vi "Gyro Steer.vi"(6 "reinitialize? (F)":bool, 10 "Target Angle":dbl) -> (0 "In Range?":bool, 2 "Steering Out":dbl format="%.2f")   [LabVIEW 2013]
uses:
  Common Code/Change Detect Boolean.vi
  Common Code/Change Detect Double.vi
  Robot Global Data.vi
  <vilib>/addons/control/pid/pid.llb/PID (DBL).vi
  <vilib>/Rock Robotics/WPI/Gyro/WPI_GyroRefNum Registry Get.vi
  <vilib>/Rock Robotics/WPI/Gyro/WPI_GyroGetAngle.vi
  <vilib>/addons/control/pid/NI_PID_pid.lvlib
panel:
  out "PID Output Range":cluster{"output high":dbl, "output low":dbl}
  out "Gyro Angle":dbl
  out "PID Gains":T1
  out "Gyro Error":dbl
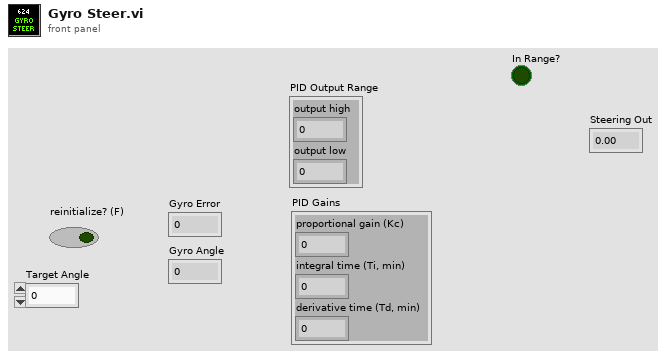
[diagram p1: front panel]
types:
  T1 = cluster{"proportional gain (Kc)":dbl, "integral time (Ti, min)":dbl, "derivative time (Td, min)":dbl}
  T2 = typedef "Dashboard UDP Packet.ctl" = cluster{"Camera":T3, "Gyro":T4, "Encoder":T6, "Auto Shift":T7, "Auton":T8, "Drive/Ramp X":dbl, "Drive/Ramp Y":dbl, "Drive/Battery Cutoff":dbl, "Pressure/Compressor Min Voltage":dbl, "Pressure/Compressor Delay":dbl, "Controller/Strafe Correction":bool, "Shooter":T9, "Rollers":T10, "Abort":bool, "Finish":bool, "IR Halo Sustain Time":dbl, "Disable Compressor":bool, "Center Omni Drive Delay":i32}
  T3 = typedef "Camera Controls.ctl" = cluster{"Camera/View Angle X":dbl, "Camera/Goal Track Timeout":dbl, "Camera/View Angle Y":dbl, "Camera/Goal Exposure":dbl, "Camera/Vision Receive Timeout":dbl, "Camera/Offset 1":dbl, "Camera/Offset 2":dbl}
  T4 = typedef "Gyro Controls.ctl" = cluster{"Gyro/Angle Tolerance":dbl, "Gyro/Steer Closeness Threshold":dbl, "Steer PID":T5, "Steer Close PID":T5}
  T5 = typedef "PID Params.ctl" = cluster{"max":dbl, "min":dbl, "P":dbl, "I":dbl, "D":dbl}
  T6 = typedef "Encoder Controls.ctl" = cluster{"Encoders/Reset":bool, "Encoders/Omni Constant":dbl, "Encoders/Omni Tick Constant":dbl, "Encoders/Left Constant":dbl, "Encoders/Right Constant":dbl, "Encoders/Right Tick Constant":dbl}
  T7 = typedef "Auto Shift Controls.ctl" = cluster{"AutoShift/Upshift Throttle Accel":dbl, "AutoShift/Speed Threshold":dbl, "AutoShift/Upshift Throttle":dbl, "AutoShift/Upshift Accel":dbl, "AutoShift/Downshift Accel":dbl, "AutoShift/Downshift Throttle":dbl, "AutoShift/Delay":dbl, "AutoShift/Enabled":bool}
  T8 = typedef "Auton Controls.ctl" = cluster{"Auton/Left Shoot X-Coord":dbl, "Auton/Right Shoot X-Coord":dbl, "DistDrive/Distance Stop Threshold":dbl, "DistDrive/Max Stop Speed":dbl, "Auton/Back Piston Time":dbl, "Auton/Manual Hot":bool, "Auton/Manual Hot Right":bool, "Default X PID":T5, "Default Y PID":T5}
  T9 = typedef "Shooter Controls.ctl" = cluster{"Shooter/Reset Time":dbl, "Shooter/Release Delay":dbl, "Shooter/Pressure Steady Time":dbl, "Shooter/Misfire Delay":dbl, "Shooter/Ball Settle Time":dbl, "Shooter/Line IR Delay":dbl, "Pressure/Upper PSI Time":dbl, "Pressure/Lower PSI Time":dbl, "Shooter/Punch Delay":dbl, "Shooter/Target Pressure":dbl, "Pressure/Line B":dbl, "Pressure/Line M":dbl, "Pressure/Shooter M":dbl, "Pressure/Shooter B":dbl, "Halo Time":dbl, "Soft Release Delay":dbl, "Soft Unpin Delay":dbl, "Soft Shoot Delay":dbl}
  T10 = typedef "Roller Controls.ctl" = cluster{"Roller/Load IRs Verify Time":dbl, "Roller/Center IR Latch Time":dbl, "Roller/Speed Front":dbl, "Roller/Speed Back":dbl, "Roller/Entry Timeout":dbl, "Roller/To Center Timeout":dbl, "Roller/Sustain Time":dbl, "Roller/Verify Center Time":dbl}
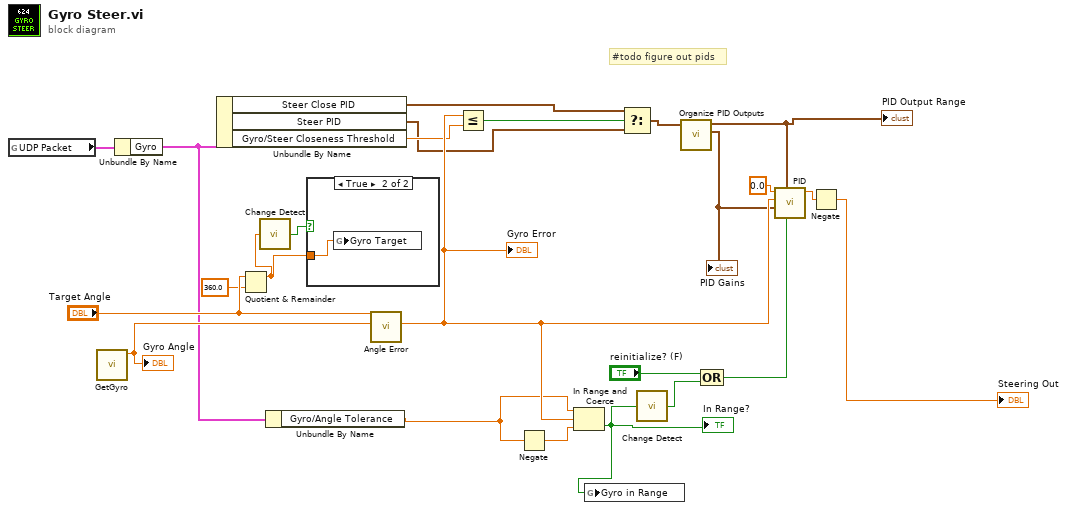
[diagram p0: block diagram]
diagram:
  # "#todo figure out pids"
  n1 = global read "Robot Global Data.vi" "UDP Packet"() -> (w9:T2)
  n2 = call "GetGyro.vi"() -> ("Angle"=w15:dbl)  [unwired: 9 in, 2 out]
  "Gyro Angle" <- w15
  n3 = Unbundle By Name(w9) -> ("Gyro"=w7:T4)
  n4 = Unbundle By Name(w7) -> ("Steer Close PID"=w5:T5, "Steer PID"=w4:T5, "Gyro/Steer Closeness Threshold"=w8:dbl)
  n5 = Quotient & Remainder(x="Target Angle", y=360.0) -> (x-y*floor(x/y)=w18:dbl)  [unwired: 1 out]
  n6 = call-poly "Change Detect.vi"("In"=w18) -> ("Changed?"=w16:bool)
  n7 = Unbundle By Name(w7) -> ("Gyro/Angle Tolerance"=w6:dbl)
  n8 = case shown="True" w16 {
    tunnel: w18 -> [_ w25]
    frame False {
    }
    frame True {
      n9 = global write "Robot Global Data.vi" "Gyro Target"(w25) -> ()
    }
  }
  n10 = call "Angle Error.vi"("Angle"=w15, "Target Angle"="Target Angle") -> ("Error"=w14:dbl)  [unwired: 9 in]
  "Gyro Error" <- w14
  n11 = Less Or Equal?(x=w14, y=w8) -> (x <= y?=w13:bool)
  n12 = Negate(x=w6) -> (-x=w22:dbl)
  n13 = In Range and Coerce(upper limit=w6, x=w14, lower limit=w22) -> (In Range?=w17:bool)  [unwired: 1 out]
  "In Range?" <- w17
  n14 = global write "Robot Global Data.vi" "Gyro in Range"(w17) -> ()
  n15 = Select(t=w5, s=w13, f=w4) -> (s? t:f=w3:T5)
  n16 = call-poly "Change Detect.vi"("In"=w17) -> ("Changed?"=w12:bool)
  n17 = call "Organize PID Outputs.vi"("PID"=w3) -> ("Gains"=w2:cluster{"P":dbl, "I":dbl, "D":dbl}, "Output Range"=w1:cluster{"max":dbl, "min":dbl})  [unwired: 9 in]
  "PID Gains" <- w2
  "PID Output Range" <- w1
  n18 = Compound Arithmetic op=OR("reinitialize? (F)", w12) -> (w10:bool)
  n19 = call-poly <vilib>:"PID.vi"("reinitialize? (F)"=w10, "output range"=w1, "PID gains"=w2, "process variable"=w14, "setpoint"=0.0) -> ("output"=w23:dbl)  [unwired: 5 in, 1 out]
  n20 = Negate(x=w23) -> (-x=→"Steering Out":dbl)
